vi "DisplayAndLogZ.vi"(0 "Log file":path=path "nologfile", 2 "message":string, 3 "action (0: log+display)":u16(ring) items=["to file + screen", "to file", "to screen", "clear screen"]) -> (7 "display":string)   [LabVIEW 2016]
doc: "This subroutine writes messages to a log file and/or to a display window. The action input has the following options:\n 0 Write message to file and display window\n 1 Write to file only\n 2 Write to display window only\n 3 Clear display window; write message to file and window\nThe log file write is omitted if the log file name equals the name shown in the \"skip file write\" field on the front panel (nologfile)."
panel:
  in  "Skip file write":path=path "nologfile"
  out "error out":errorcluster
  in  "error in (no error)":errorcluster
  # "Program constants"
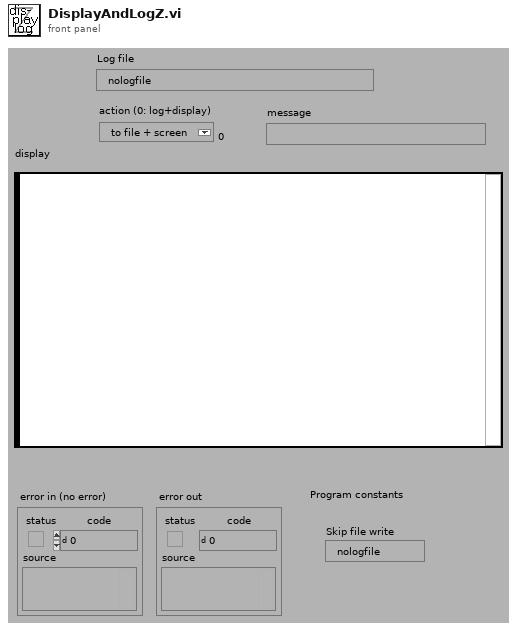
[diagram p1: front panel]
types:
  T1 = enum16{"open", "open or create", "create or replace", "create"}
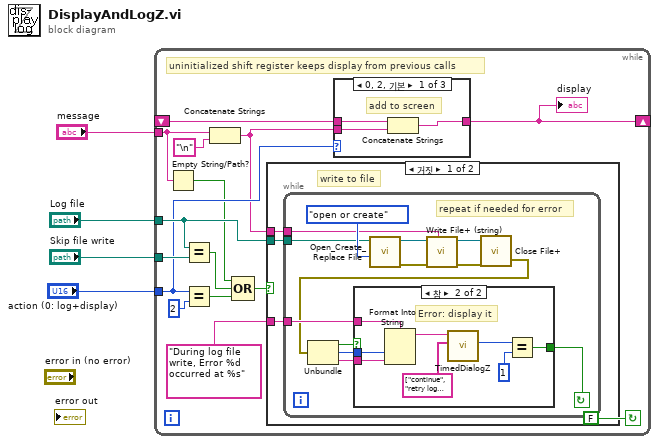
[diagram p0: block diagram]
diagram:
  n1 = while {
    tunnel: "Skip file write" -> [w17]
    tunnel: "action (0: log+display)" -> [w14]
    tunnel: "Log file" -> [w18]
    tunnel: "message" -> [w8]
    shift-left: _ -> [w19]
    shift-right: [w6] -> _
    stop <- FALSE continue-if-true
    # "uninitialized shift register keeps display from previous calls"
    n2 = Empty String/Path?(string/path=w8) -> (empty?=w10:bool)
    n3 = Equal?(x=w18, y=w17) -> (x = y?=w11:bool)
    n4 = Equal?(x=w14, y=u16 2 ("t")) -> (x = y?=w12:bool)
    n5 = Concatenate Strings(w8, "\n" ("Substring")) -> (w7:string)
    n6 = Compound Arithmetic op=OR(w10, w11, w12) -> (w9:bool)
    n7 = case shown="거짓" w9 {
      tunnel: w7 -> [w22 _]
      tunnel: w18 -> [w21 _]
      tunnel: "During log file write, Error %d occurred at %s" -> [w20 _]
      frame False {
        # "write to file"
        n8 = while {
          tunnel: w20 -> [w24]
          tunnel: w21 -> [w29]
          tunnel: w22 -> [w30]
          stop <- w27 continue-if-true
          # "repeat if needed for error"
          n9 = call <vilib>:"Open_Create_Replace File.vi"("function (open:0)"=T1."open or create", "file path"=w29) -> ("error out"=w31:errorcluster, "refnum"=w34:refnum<file>)  [unwired: 6 in, 2 out]
          n10 = call <vilib>:"Write File+ (string).vi"("string"=w30, "error in (no error)"=w31, "refnum"=w34) -> ("error out"=w32:errorcluster, "dup refnum"=w33:refnum<file>)  [unwired: 4 in, 1 out]
          n11 = call <vilib>:"Close File+.vi"("error in (no error)"=w32, "refnum"=w33) -> ("error out"=w23:errorcluster)  [unwired: 3 in, 2 out]
          n12 = Unbundle(w23) -> ("status"=w28:bool, "code"=w26:i32, "source"=w25:string)
          n13 = case shown="참" w28 {
            selector: w28 -> [w36 _]
            tunnel: w24 -> [_ w44]
            tunnel: [w36 w39] -> w27
            tunnel: w26 -> [_ w38]
            tunnel: w25 -> [_ w37]
            frame False {
              # "No error"
            }
            frame True {
              # "Error: display it"
              n14 = Format Into String(format string=w44, w38, w37) -> (resulting string=w43:string)  [unwired: 2 in, 1 out]
              n15 = call "TimedDialogZ.vi"("option list"=string[] ["continue", "retry log write"], "Dialog text"=w43) -> ("selection (timeout -1)"=w41:i32)  [unwired: 7 in]
              n16 = Equal?(x=w41, y=1) -> (x = y?=w39:bool)
            }
          }
        }
      }
      frame True {
        # "No file write"
      }
    }
    n17 = case shown="0, 2, 기본" w14 {
      tunnel: w19 -> [w47 w48 _]
      tunnel: w7 -> [w46 _ w49]
      tunnel: [w45 w48 w49] -> w6
      frame 0, 2, Default {
        # "add to screen"
        n18 = Concatenate Strings(w47, w46) -> (w45:string)
      }
      frame 1 {
        # "skip screen"
      }
      frame 3 {
        # "clear screen"
      }
    }
    "display" <- w6
  }
